vi "Read Attributes.vi"(11 "Start Test Msg":refnum<class "Start Test Msg.lvclass">) -> (2 "Payload":cluster{"Selected Tests":string[]})   [LabVIEW 2017, in "User Interface.lvlib" / "Start Test Msg.lvclass"]
uses:
  Start Test Msg.lvclass
  Start Test Msg.lvclass/Start Test Msg.ctl
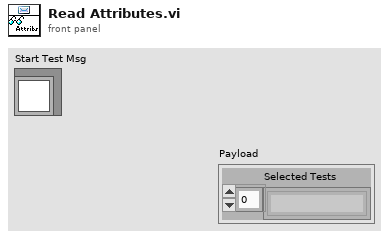
[diagram p1: front panel]
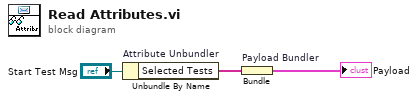
[diagram p0: block diagram]
diagram:
  n1 = Unbundle By Name "Attribute Unbundler"("Start Test Msg") -> ("Selected Tests"=w1:string[])
  n2 = Bundle "Payload Bundler"("Selected Tests"=w1) -> (→"Payload":cluster{"Selected Tests":string[]})  [unwired: 1 in]
